vi "Get (Boolean).vi"(10 "Key":string, 11 "Dictionary in":variant) -> (1 "value":bool, 2 "found":bool, 3 "Dictionary out":variant)   [LabVIEW 2013, in "Dictionary.lvlib"]
doc: "Gets (Read) value for the passed in key."
uses:
  Dictionary.lvlib
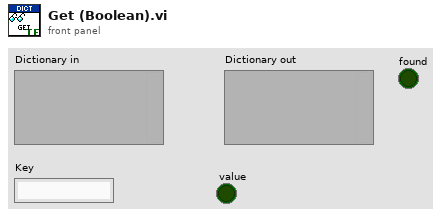
[diagram p1: front panel]
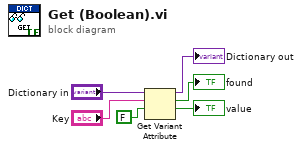
[diagram p0: block diagram]
diagram:
  n1 = Get Variant Attribute(Variant="Dictionary in", name="Key", default value (empty Variant)=FALSE) -> (duplicate Variant=→"Dictionary out":variant, found=→"found":bool, value=→"value":bool)  [unwired: 1 in, 1 out]
